vi "例程14-提取指定的波形数据.vi"() -> ()   [LabVIEW 2016]
uses:
  <vilib>/Waveform/WDTOps.llb/WDT Index Channel DBL.vi
  <vilib>/measure/NI_MABase.lvlib
panel:
  out "索引波形图":waveform(dbl)(graph)
  out "波形图":dynamicdata(graph)
  out "波形数据数组":waveform(dbl)[](array[waveform])
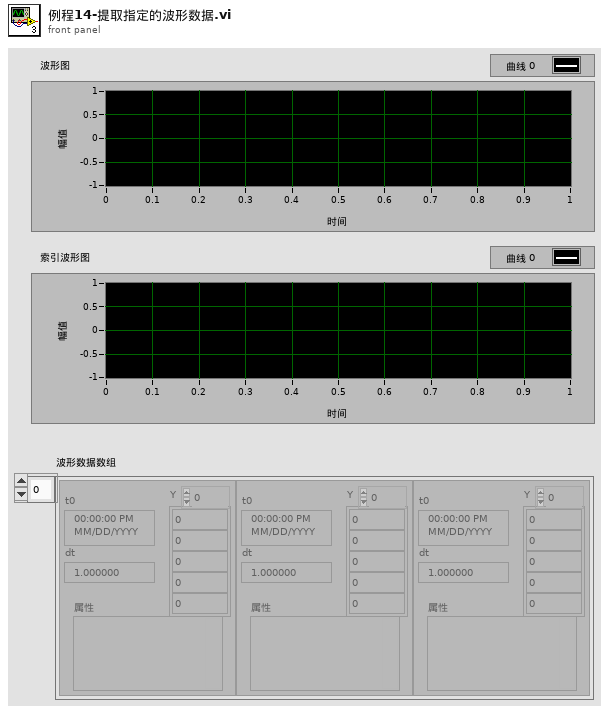
[diagram p1: front panel]
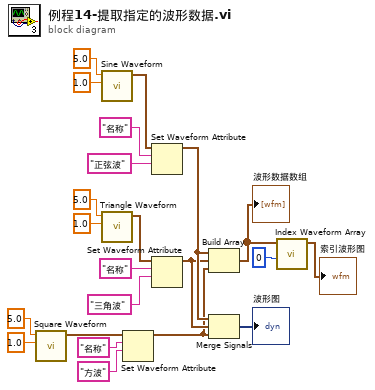
[diagram p0: block diagram]
diagram:
  n1 = call <vilib>:"Square Waveform.vi"("amplitude"=1.0, "frequency"=5.0) -> ("signal out"=w14:waveform(dbl))  [unwired: 8 in, 1 out]
  n2 = call <vilib>:"Sine Waveform.vi"("amplitude"=1.0, "frequency"=5.0) -> ("signal out"=w16:waveform(dbl))  [unwired: 8 in, 1 out]
  n3 = call <vilib>:"Triangle Waveform.vi"("amplitude"=1.0, "frequency"=5.0) -> ("signal out"=w15:waveform(dbl))  [unwired: 8 in, 1 out]
  n4 = Set Waveform Attribute(5:"方波", 6:"名称" ("名称"), 7:w14) -> (3:w3:waveform(dbl))  [unwired: 1 in, 2 out]
  n5 = Set Waveform Attribute(5:"正弦波" ("名称"), 6:"名称" ("名称"), 7:w16) -> (3:w5:waveform(dbl))  [unwired: 1 in, 2 out]
  n6 = Set Waveform Attribute(5:"三角波", 6:"名称" ("名称"), 7:w15) -> (3:w4:waveform(dbl))  [unwired: 1 in, 2 out]
  n7 = Build Array(w5, w4, w3) -> (w9:waveform(dbl)[])
  "波形数据数组" <- w9
  n8 = Merge Signals(w5, w4, w3) -> (→"波形图":dynamicdata)
  n9 = call-poly <vilib>:"Index Waveform Array.vi"("index"=0, "waveform array"=w9) -> ("waveform"=→"索引波形图":waveform(dbl))  [unwired: 8 in, 1 out]
